vi "JSON Scalar Probe.vi"(11 "JSON Scalar In":refnum<class "JSON Scalar.lvclass">) -> (2 "Value String":string, 3 "Boolean":bool)   [LabVIEW 2011, in "JSON Scalar.lvclass"]
uses:
  JSON Scalar.lvclass
panel:
  out "JSON":string
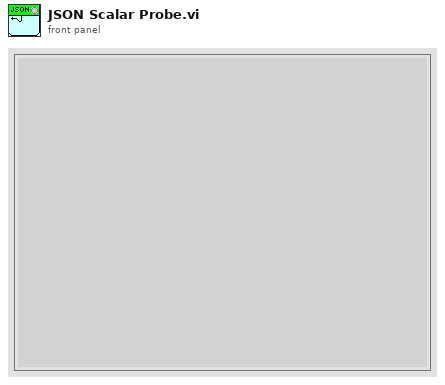
[diagram p1: front panel]
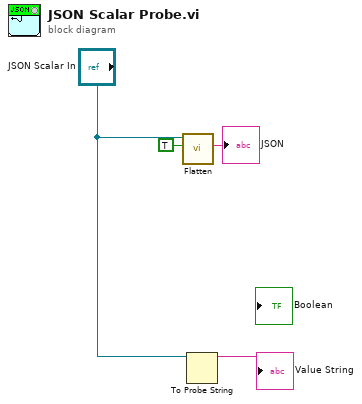
[diagram p0: block diagram]
diagram:
  n1 = call-dynamic "Flatten.vi"("Pretty Print?"=TRUE, "JSON Scalar in"="JSON Scalar In") -> ("String"=→"JSON":string)  [unwired: 8 in, 1 out]
  n2 = To Probe String(7:"JSON Scalar In") -> (3:→"Value String":string)  [unwired: 2 in, 1 out]
